vi "grabLastGrayScaleImageAttempt.vi"(4 "bufferNumberIn":u32, 5 "ImageInstance":T2, 6 "errorIn":errorcluster, 7 "SessionIn":T1) -> (0 "ImageOut":T2, 1 "errorOut":errorcluster, 2 "bufferNumberActual":u32, 3 "sessionOut":T1)   [LabVIEW 2021]
uses:
  <vilib>/vision/Image Controls.llb/IMAQ Image.ctl
  <vilib>/userdefined/High Color/IMAQdx.ctl
  <vilib>/vision/Management.llb/Cast Image 2 Method.ctl
  <vilib>/vision/driver/IMAQdx.llb/IMAQdx Buffer Number Mode.ctl
  niimaqdx.dll
  <vilib>/vision/driver/NI_Vision_Acquisition_Software.lvlib
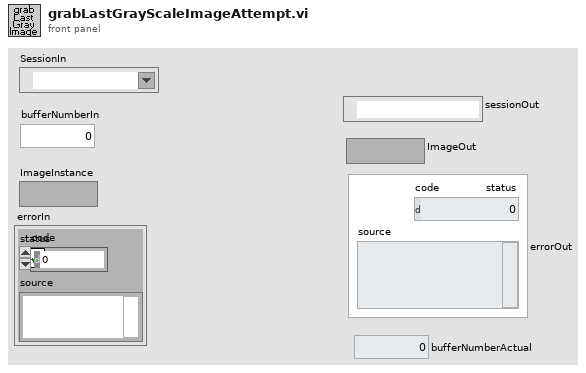
[diagram p1: front panel]
types:
  T1 = typedef "IMAQdx.ctl" = refnum<k21>
  T2 = typedef "IMAQ Image.ctl" = refnum<image>
  T3 = typedef "NI_Vision_Acquisition_Software.lvlib/IMAQdx Buffer Number Mode.ctl" = enum32{"Next", "Last", "Buffer Number", "Every", "Last New"}
  T4 = typedef "Cast Image 2 Method.ctl" = u32
  T5 = typedef "Image Type" = u32
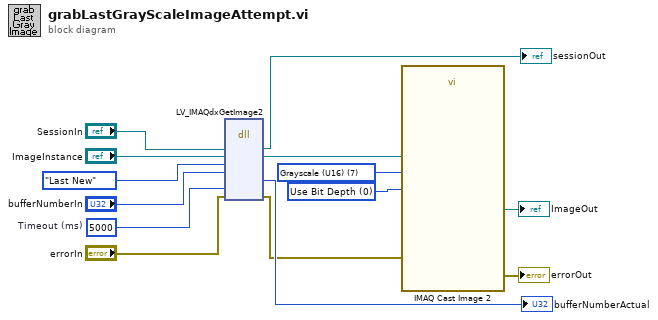
[diagram p0: block diagram]
diagram:
  w10 = 5000  # Timeout (ms)
  w13 = T4 0 items=["Use Bit Depth", "Shift", "Use Lookup Table"] ("Method")
  w12 = T5 7 items=["Grayscale (U8)", "Grayscale (I16)", "Grayscale (SGL)", "Complex (CSG)", "RGB (U32)", "HSL (U32)", "RGB (U64)", "Grayscale (U16)"] ("Image Type")
  n1 = dll-call lib="niimaqdx.dll" fn="LV_IMAQdxGetImage2"("refnum"="SessionIn", "image"="ImageInstance", "mode"=IMAQdx_Buffer_Number_Mode."Last New" ("Buffer Number Mode"), "bufferNumberDesired"="bufferNumberIn", "timeoutMs"=w10, "error"="errorIn") -> ("refnum"=→"sessionOut":T1, "image"=w2:T2, "bufferNumberActual"=→"bufferNumberActual":u32, "error"=w6:errorcluster)  [unwired: 8 in, 2 out]
  n2 = call "IMAQ Cast Image 2"("Image Src"=w2, "Method"=w13, "Image Type"=w12, "error in (no error)"=w6) -> ("Image Dst Out"=→"ImageOut":T2, "error out"=→"errorOut":errorcluster)  [unwired: 10 in]
